vi "Create_New_Video_File.vi"(2 "error in (no error)":errorcluster, 3 "Codec":string, 4 "AVI Refnum IN":T1) -> (0 "error out":errorcluster, 1 "AVI Refnum OUT":T1)   [LabVIEW 2010]
uses:
  <vilib>/vision/Avi.llb/IMAQ AVI2 Refnum.ctl
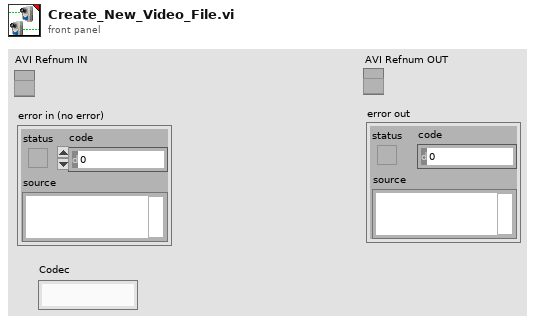
[diagram p1: front panel]
types:
  T1 = typedef "IMAQ AVI2 Refnum.ctl" = refnum<k20>
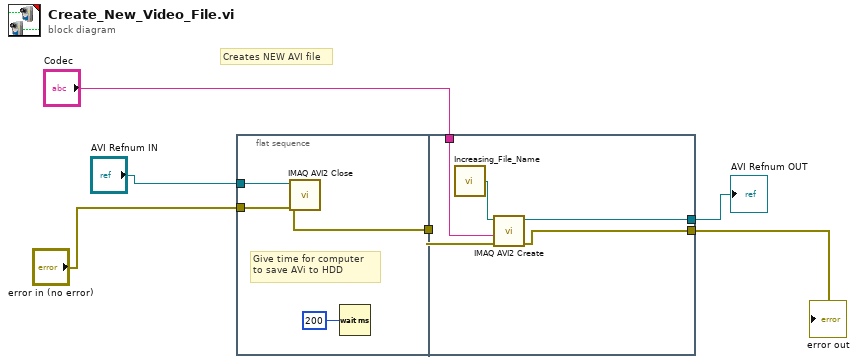
[diagram p0: block diagram]
diagram:
  # "Creates NEW AVI file"
  n1 = flat-sequence {
    tunnel: [w10] -> w6
    tunnel: "AVI Refnum IN" -> [w8]
    tunnel: "error in (no error)" -> [w7]
    tunnel: w6 -> [w12]
    tunnel: [w15] -> w3
    tunnel: [w14] -> w4
    tunnel: "Codec" -> [w11]
    frame #0 {
      # "Give time for computer \nto save AVi to HDD"
      n2 = call "IMAQ AVI2 Close"("error in (no error)"=w7, "AVI Refnum"=w8) -> ("error out"=w10:errorcluster)  [unwired: 9 in]
      n3 = Wait (ms)(milliseconds to wait=u32 200) -> ()  [unwired: 1 out]
    }
    frame #1 {
      n4 = call "Increasing_File_Name.vi"() -> ("Final AVI path"=w13:path)  [unwired: 1 in]
      n5 = call "IMAQ AVI2 Create"("error in (no error)"=w12, "Codec"=w11, "AVI Path"=w13) -> ("error out"=w15:errorcluster, "AVI Refnum"=w14:T1)  [unwired: 7 in]
    }
  }
  "AVI Refnum OUT" <- w4
  "error out" <- w3
